vi "TimedReadFromTextFile.vi"() -> ()   [LabVIEW 2022 SP3]
uses:
  <vilib>/Platform/TimedLoop/XDataNode/timing_clust.ctl
  <vilib>/Platform/TimedLoop/XDataNode/nitl_modes.ctl
  <vilib>/Platform/TimedLoop/XDataNode/wakeup.ctl
  <vilib>/Platform/TimedLoop/scheduler/LVUserAPI/_suppVIs/Create_1kHz_TSource.vi
  <vilib>/platform/TimedLoop/XDataNode/XDataNode.xnode
  <vilib>/Platform/TimedLoop/XDataNode/XDNodeRunTimeDep.lvlib
panel:
  in  "Sample Rate (kHz)":i64
  in  "stop 2":bool
  out "Waveform Chart 2":dbl(graph)
  out "offset (in bytes) 2":i64
  out "output waveform":waveform(dbl)
  out "Search Pattern":string
  in  "Separator":string="."
  in  "Delimiter":string="\t"
  in  "Skip Lines":i32=21
  in  "Path":path=path "C:/Users/LAV-UFSC/Desktop/acc_time/Previous Data/handlebar_acc1_run1.txt"
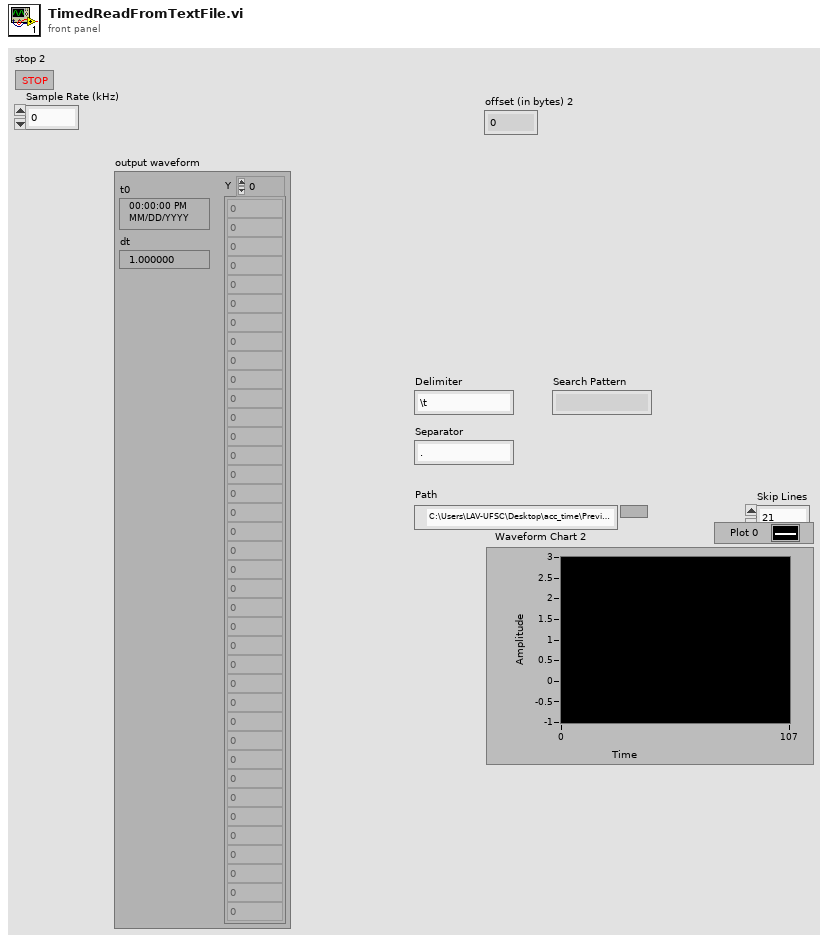
[diagram p1: front panel]
types:
  T1 = enum16{"open", "replace", "create", "open or create", "replace or create", "replace or create with confirmation"}
  T2 = typedef "XDNodeRunTimeDep.lvlib/timing_clust.ctl" = cluster{"Expected End [f-1]":u64, "Actual End [f-1]":u64, "Finished Late? [f-1]":bool, "Expected End [i-1]":u64, "Actual End [i-1]":u64, "Finished Late? [i-1]":bool, "Expected Start [i]":u64, "Actual Start [i]":u64, "Expected Start [f]":u64, "Actual Start [f]":u64, "Source Name":string, "Structure Name":string, "Period":i64, "Deadline":i64, "Offset":i64, "Start":i64, "Priority":i32, "Timeout":i32, "Mode":T3, "Wakeup Reason":T4, "Error":errorcluster, "Source Type":string, "Secondary Source Type":string, "Global End Time":u64, "Global Start Time":u64, "Frame Duration":u64, "Iteration Duration":u64, "Assigned CPU":i32, "I/O Scan Engine Mode":u32}
  T3 = typedef "XDNodeRunTimeDep.lvlib/nitl_modes.ctl" = enum32{"No Change", "Process missed periods, maintain original phase", "Discard missed periods, maintain original phase", "Process missed periods, ignore original phase", "Discard missed periods, ignore original phase"}
  T4 = typedef "XDNodeRunTimeDep.lvlib/wakeup.ctl" = enum32{"Normal", "Aborted", "Asynchronous wakeup", "Timing source error", "Timed loop error", "Timeout"}
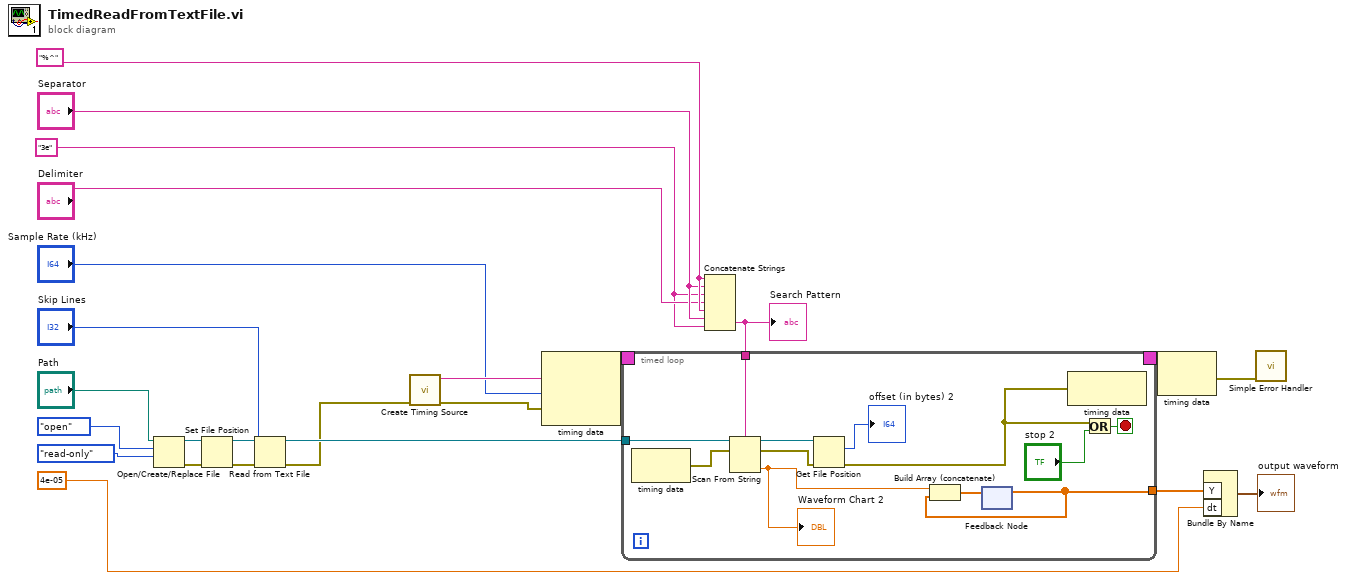
[diagram p0: block diagram]
diagram:
  w14 = "3e" ("string")
  w19 = "%^" ("format string")
  n1 = Open/Create/Replace File(file path (use dialog)="Path", operation (0:open)=T1."open", access (0:read/write)=enum16{"read/write", "read-only", "write-only"}."read-only") -> (refnum out=w15:refnum<file>, error out=w23:errorcluster)  [unwired: 3 in, 1 out]
  n2 = Set File Position(refnum=w15, error in=w23) -> (refnum out=w16:refnum<file>, error out=w4:errorcluster)  [unwired: 2 in]
  n3 = Read from Text File(file (use dialog)=w16, count="Skip Lines", error in=w4) -> (refnum out=w3:refnum<file>, error out=w2:errorcluster)  [unwired: 1 in, 2 out]
  n4 = call-poly <vilib>:"Create Timing Source.vi"("error in (no error)"=w2) -> ("error out"=w8:errorcluster, "name (out)"=w9:string)  [unwired: 9 in]
  n5 = node-c288(w9, "Sample Rate (kHz)", w8) -> (w11:T2)
  n6 = Concatenate Strings(w19, "Separator", w14, "Delimiter", w19, "Separator", w14) -> (w5:string)
  "Search Pattern" <- w5
  n7 = timed-loop {
    timing: w11 -> [_]
    timing-out: [_] -> w10
    tunnel: [w30] -> w7
    tunnel: w5 -> [w29]
    tunnel: w3 -> [w28]
    stop <- w31 stop-if-true
    n8 = node-c288() -> (w27:errorcluster)  [unwired: 1 in]
    n9 = Scan From String(w29, w28, w27) -> (w36:refnum<file>, w35:errorcluster, output 2=w33:dbl)  [unwired: 3 in]
    "Waveform Chart 2" <- w33
    n10 = Get File Position(4:w35, 7:w36) -> (0:w26:errorcluster, 2:→"offset (in bytes) 2":i64)  [unwired: 1 out]
    n11 = feedback #1() -> (w30:dbl[])  [unwired: 1 in]
    n12 = Build Array (concatenate)(w33, w30) -> (w32:dbl[])
    n13 = feedback-in #1(w32) -> ()
    n14 = node-c288(w26) -> ()  [unwired: 1 out]
    n15 = Or(x=w26, y="stop 2") -> (x .or. y?=w31:bool)
  }
  n16 = node-c288(w10) -> (w6:errorcluster)
  n17 = Bundle By Name("Y"=w7, "dt"=4e-05) -> (→"output waveform":waveform(dbl))  [unwired: 1 in]
  n18 = call <vilib>:"Simple Error Handler.vi"("error in (no error)"=w6) -> ()  [unwired: 4 in, 5 out]
